vi "ReversedEngineering GetCompleteDependencyInfo.vi"(1 "path":path[](array[path]), 2 "SearchElements":T2[](array[typedef]), 4 "IgnoreClasses":path[](array[path]), 5 "error in (no error)":errorcluster, 6 "Only Create this class and its dependencis":bool, 7 "SyncOption":T1, 8 "Only analyse this class methods and attributes(False)":bool, 10 "CreateApplicationNode":bool) -> (15 "classInfos":T7[](array[typedef]), 16 "TypeDefs":T3[](array[typedef]), 17 "Cancelled":bool, 19 "error out":errorcluster)   [LabVIEW 2014]
doc: "Gets current diagram values"
uses:
  <resource>/Framework/Providers/Open_GDS/UML/ReversedEngineering/ReversedEngineering ClassInfoType.ctl
  <resource>/Framework/Providers/Open_GDS/UML/UMLEditor/UMLEditor_VisibilityType.ctl
  <resource>/Framework/Providers/Open_GDS/UML/ReversedEngineering/ReversedEngineering AttributeInfoType.ctl
  <resource>/Framework/Providers/Open_GDS/ClassProviders/Common/CommonVIs/CommonVIs_AttributeDataType.ctl
  <resource>/Framework/Providers/Open_GDS/UML/ReversedEngineering/ReversedEngineering_ClassDependencyDetailsType.ctl
  <resource>/Framework/Providers/Open_GDS/ClassProviders/Common/ScriptingFunctions/SubVIs/Scripting_ViDependencyType.ctl
  <resource>/Framework/Providers/Open_GDS/UML/ReversedEngineering/ReversedEngineering TypeDefType.ctl
  <resource>/Framework/Providers/Open_GDS/UML/ReversedEngineering/ReversedEngineering RecursiveSearchElements.ctl
  <resource>/Framework/Providers/Open_GDS/UML/UMLEditor/UMLEditor_SyncOptions.ctl
  <resource>/Framework/Providers/Open_GDS/UML/UMLEditor/UMLEditor BusyDialogAction.ctl
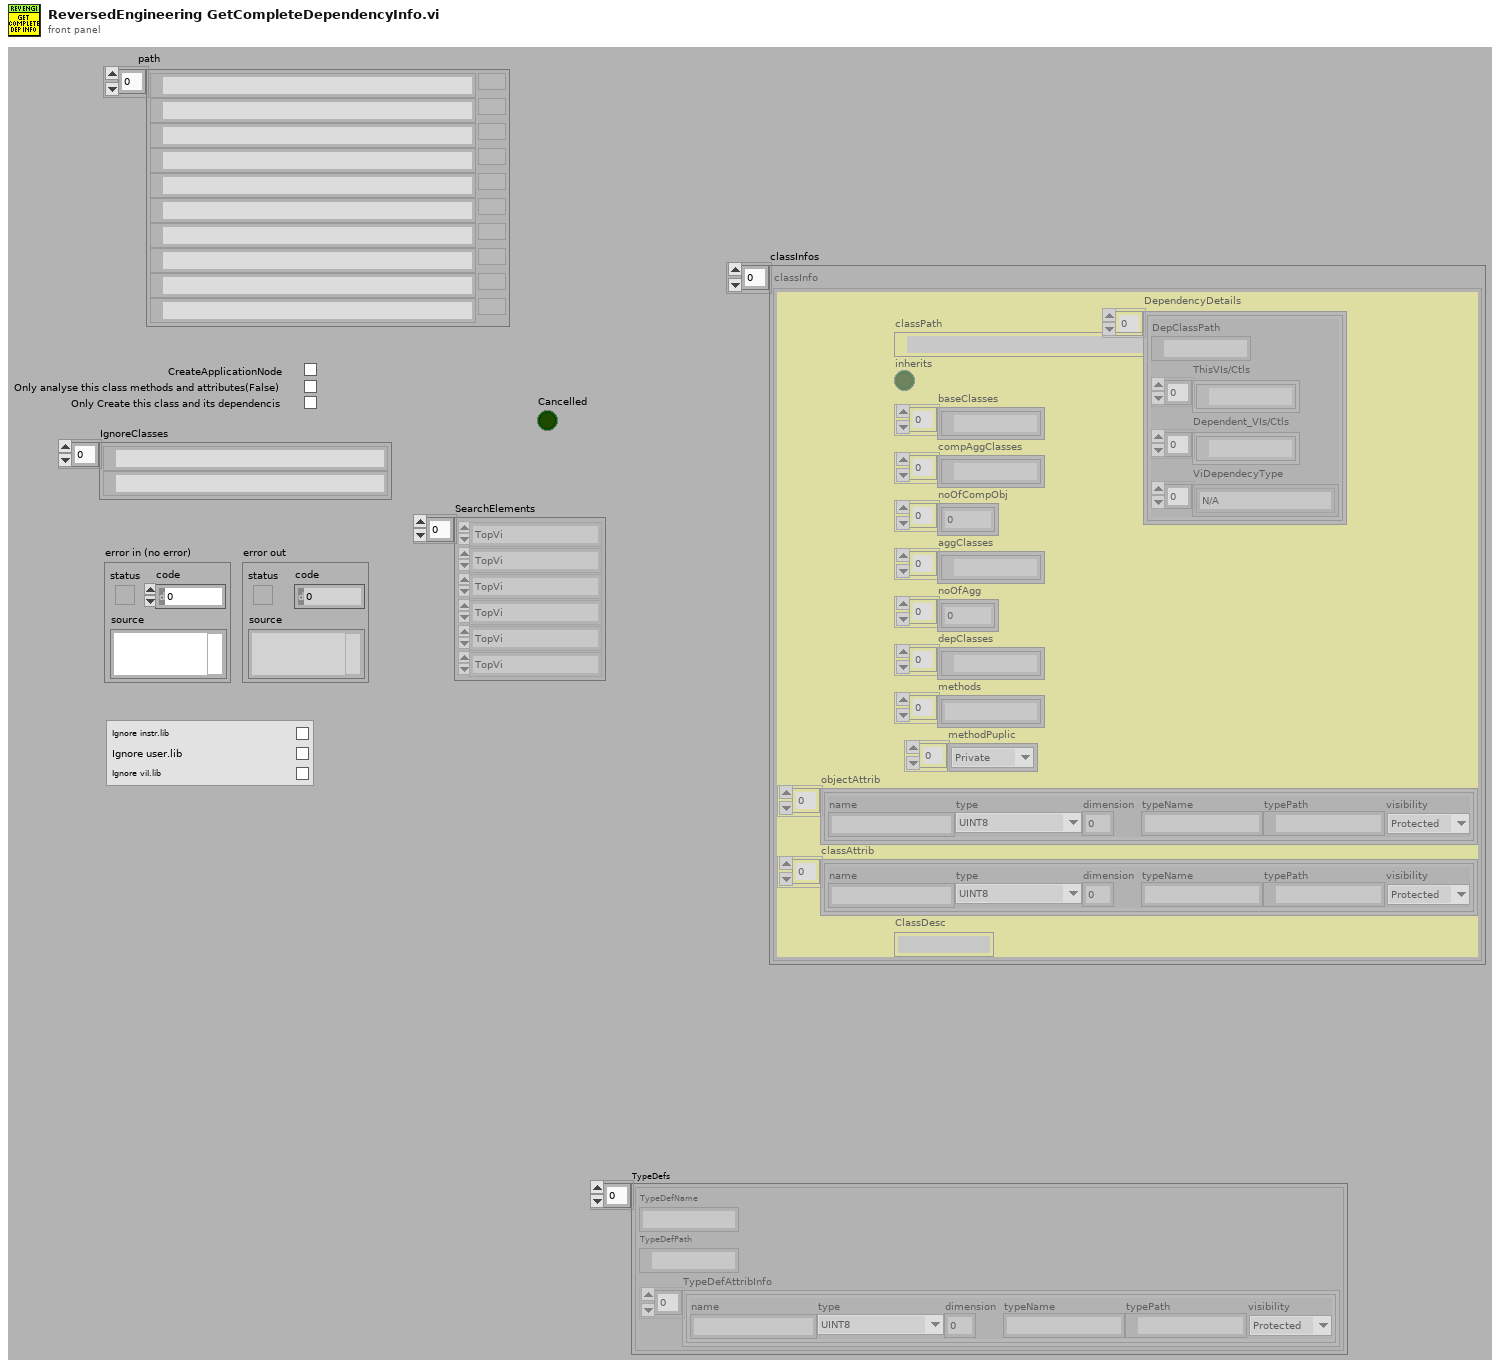
[diagram p1: front panel]
types:
  T1 = typedef "UMLEditor_SyncOptions.ctl" = cluster{"IgnoreInstrLib":bool, "IgnoreUserLib":bool, "IgnoreViLib":bool}
  T2 = typedef "ReversedEngineering RecursiveSearchElements.ctl" = enum16{"TopVi", "Class", "Dir", "Dir(rec.)"}
  T3 = typedef "ReversedEngineering TypeDefType.ctl" = cluster{"TypeDefName":string, "TypeDefPath":path, "TypeDefAttribInfo":T4[]}
  T4 = typedef "ReversedEngineering AttributeInfoType.ctl" = cluster{"name":string, "type":T5, "dimension":i32, "typeName":string, "typePath":path, "visibility":T6}
  T5 = typedef "CommonVIs_AttributeDataType.ctl" = enum16{"UINT8", "INT8", "UINT16", "INT16", "UINT32", "INT32", "UINT64", "INT64", "SGL", "DBL", "EXT", "CSG", "CDB", "CXT", "TimeStamp", "STRING", "PATH", "BOOL", "ENUM", "RefNum", "VIRefNum", "LabVIEW Class", "Cluster", "Variant", "TypeDef", "Waveform", "LabVIEW Object", "Other", "void"}
  T6 = typedef "UMLEditor_VisibilityType.ctl" = enum16{"Public", "Private", "Protected"}
  T7 = typedef "ReversedEngineering ClassInfoType.ctl" = cluster{"classPath":path, "inherits":bool, "baseClasses":path[], "compAggClasses":path[], "noOfCompObj":i32[], "aggClasses":path[], "noOfAgg":i32[], "depClasses":path[], "methods":string[], "methodPuplic":T6[], "objectAttrib":T4[], "classAttrib":T4[], "ClassDesc":string, "DependencyDetails":T8[]}
  T8 = typedef "ReversedEngineering_ClassDependencyDetailsType.ctl" = cluster{"DepClassPath":path, "ThisVIs/Ctls":path[], "Dependent_VIs/Ctls":path[], "ViDependecyType":T9[]}
  T9 = typedef "Scripting_ViDependencyType.ctl" = enum16{"N/A", "Launches"}
  T10 = cluster{"dependencyClassPath":path[], "topVIPath":path, "classInfos":T7[], "calleesVIs":path[], "VIRef":refnum<vi>[], "TypeDefs":T3[], "TopVIPath":path, "SearchOnlyClasses":bool, "SearchDirs":path[], "SearchOnlyTopVIs":bool, "lvclasses":path[]}
  T11 = enum16{"Get Library Info", "Create Library Info", "Clear Library Info"}
  T12 = typedef "UMLEditor BusyDialogAction.ctl" = enum16{"Initialize", "Open(VIs)", "Open(i)", "Send_I-Value", "SendStatusMessage", "GetBusyDialogStatus", "Close", "Quit"}
  T13 = typedef "Librarian File Info Out.ctl" = cluster{"creation date":u32, "last mod date":u32, "type":string, "creator":string, "LV version":i32, "size":i32, "top level":bool}
  T14 = typedef "Scripting_VIClassDependency.ctl" = cluster{"VIPath":path, "Class":string, "ClassPath":path, "ViDependencyType":T9}
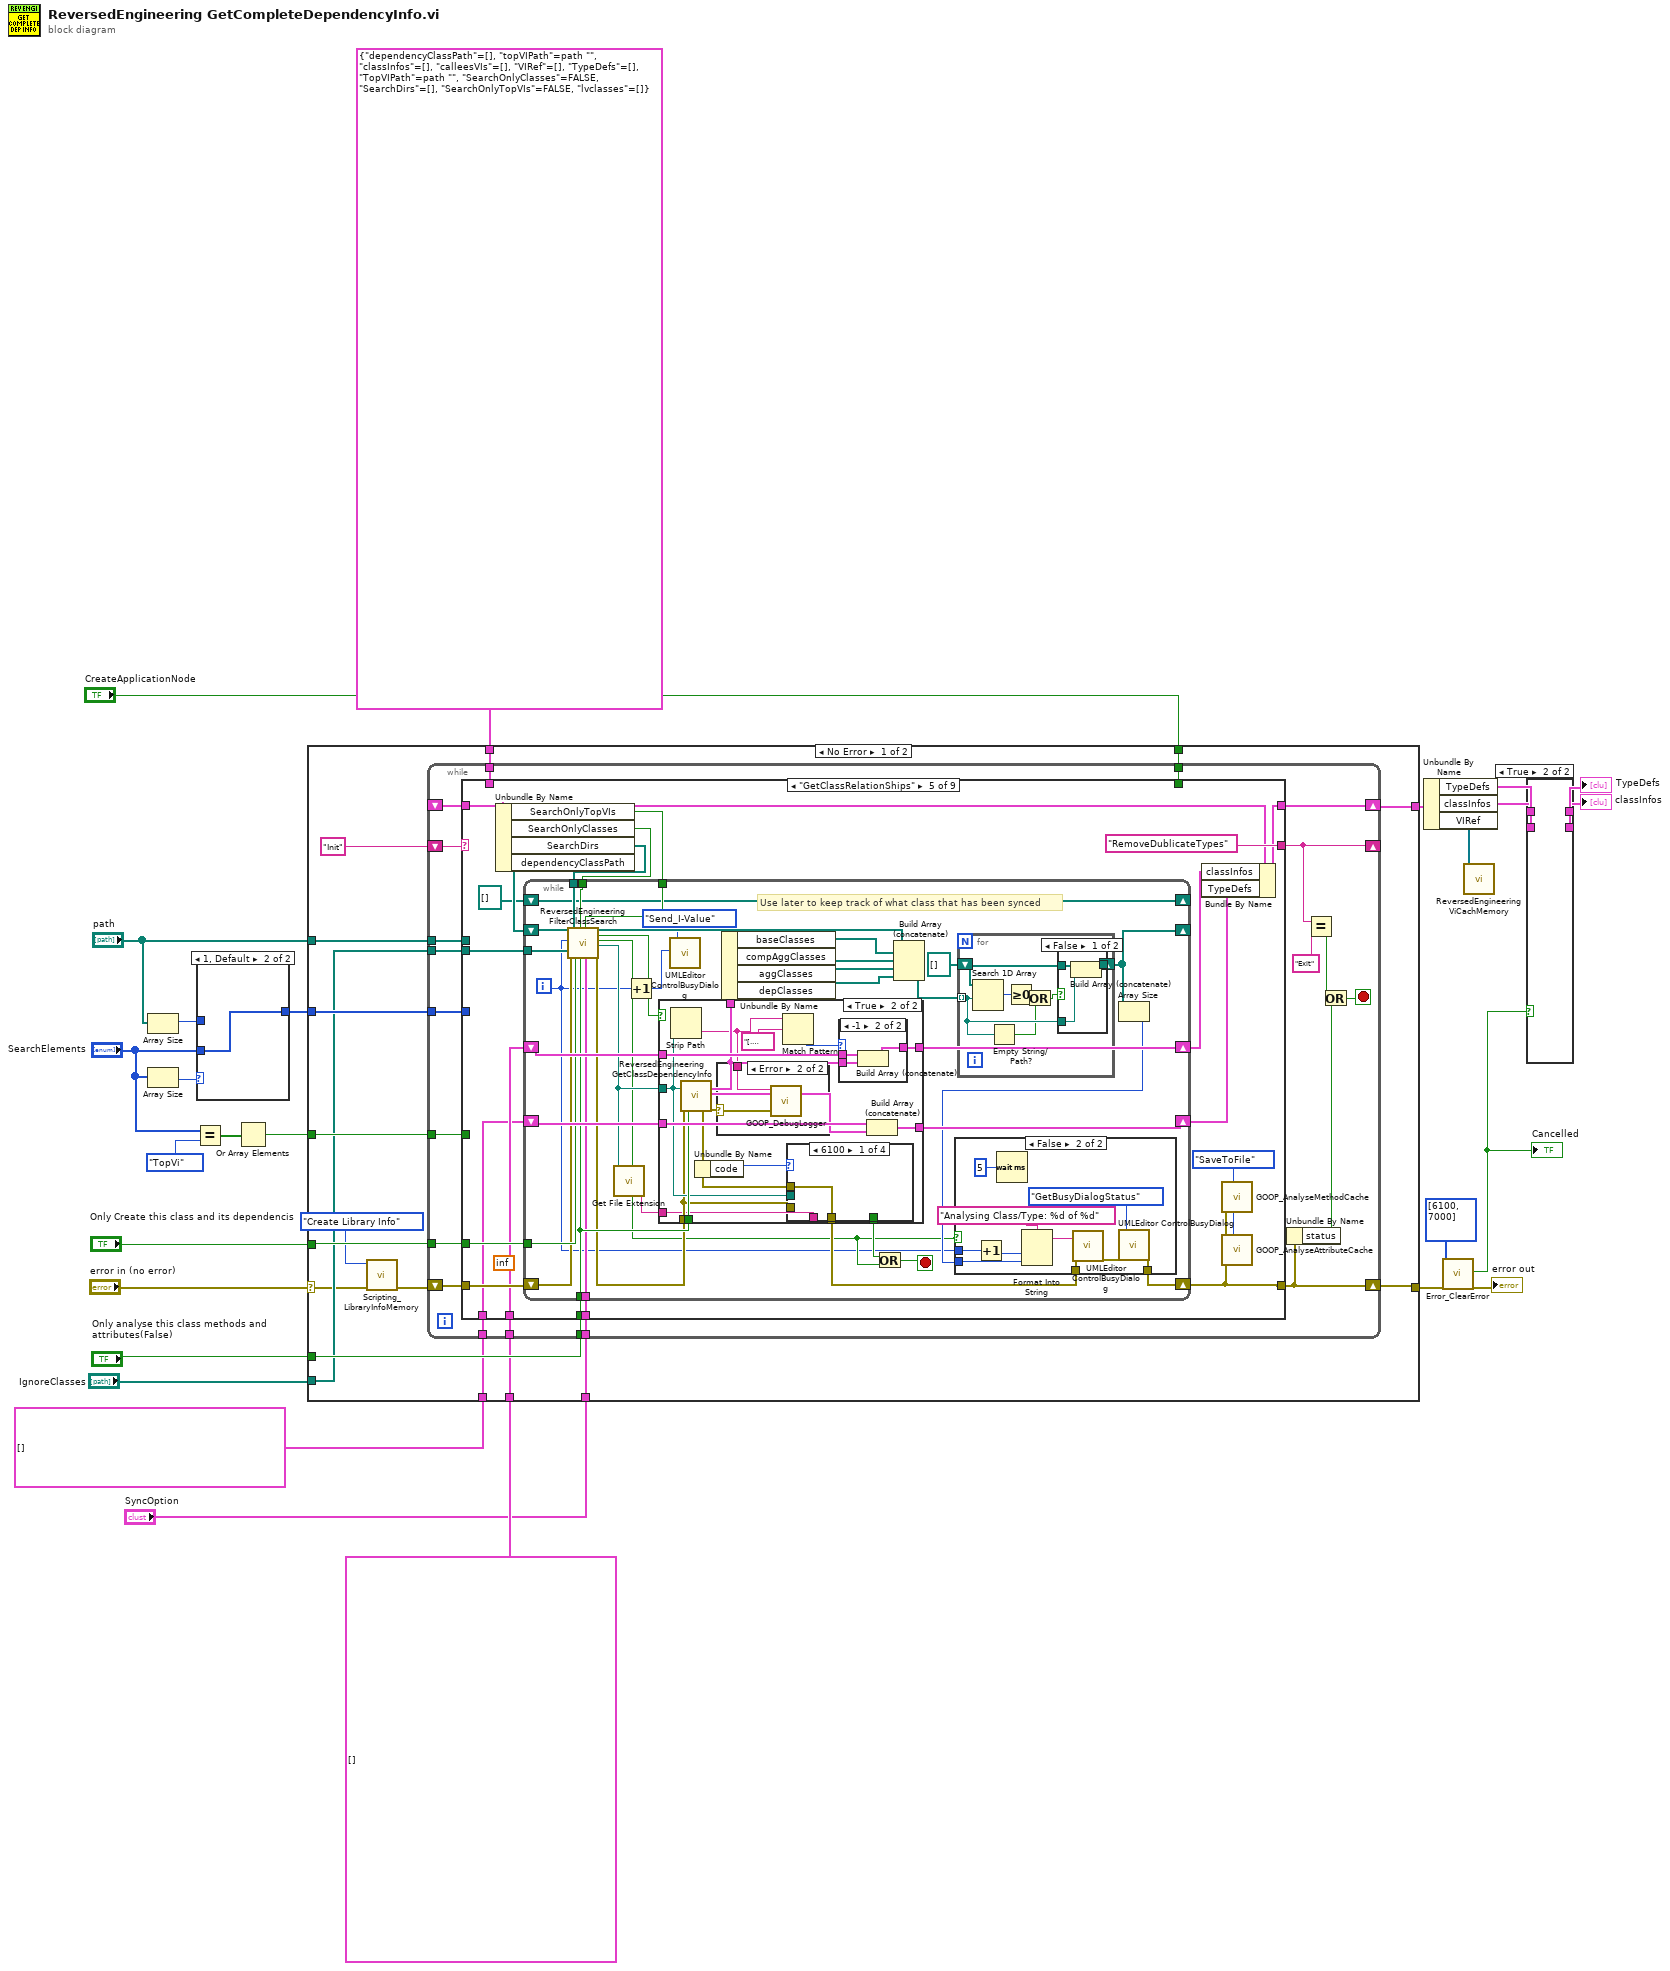
[diagram p0: block diagram]
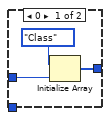
[diagram p3: hidden frame]
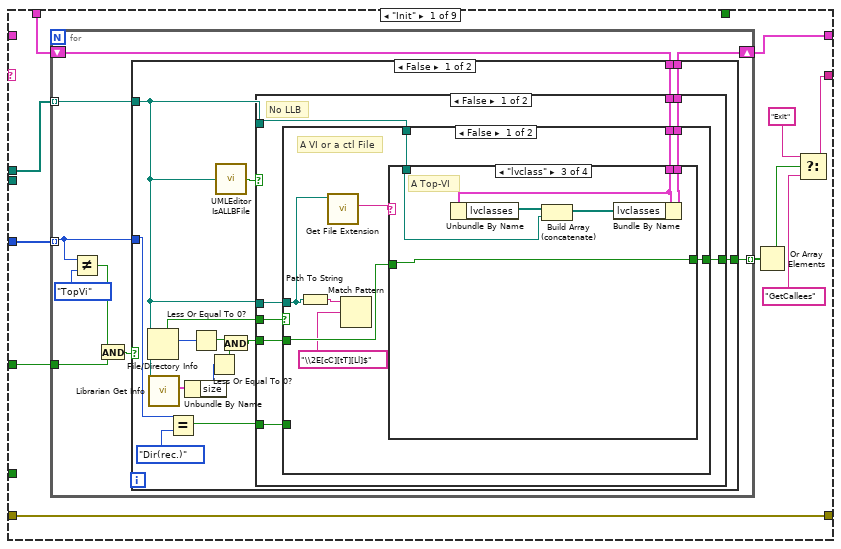
[diagram p4: hidden frame]
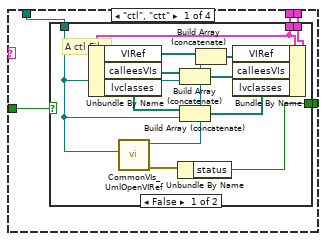
[diagram p5: hidden frame]
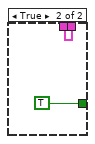
[diagram p6: hidden frame]
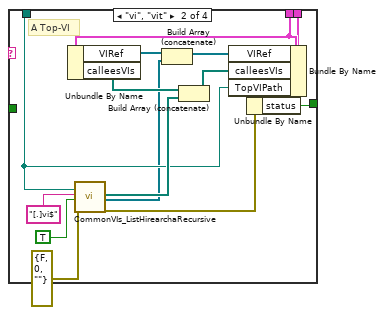
[diagram p7: hidden frame]
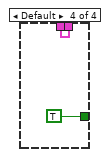
[diagram p8: hidden frame]
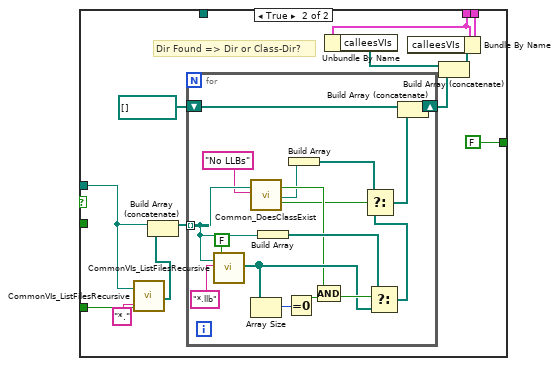
[diagram p9: hidden frame]
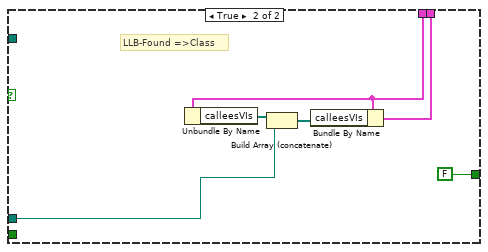
[diagram p10: hidden frame]
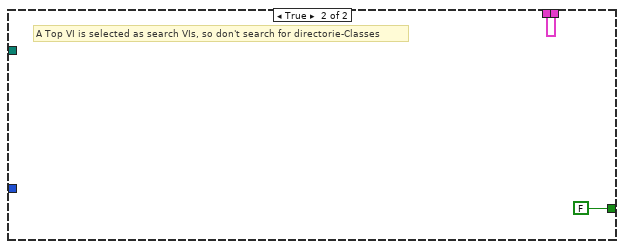
[diagram p11: hidden frame]
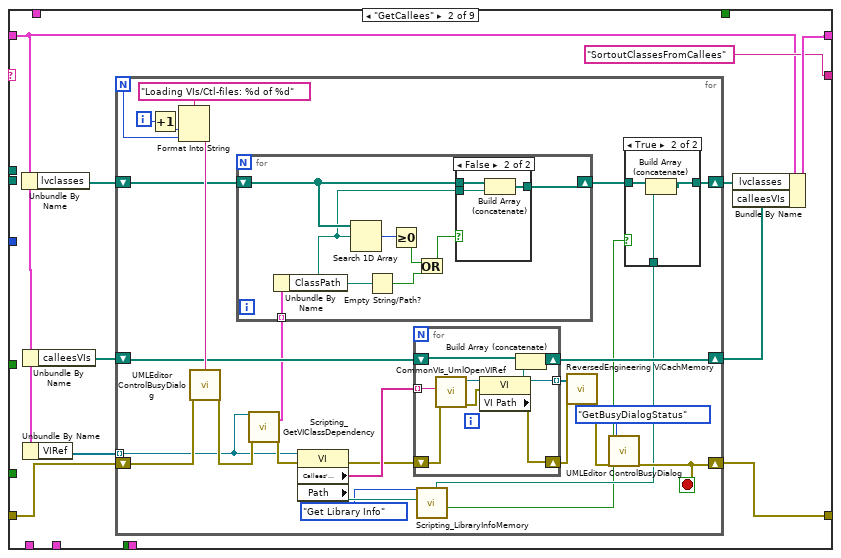
[diagram p12: hidden frame]
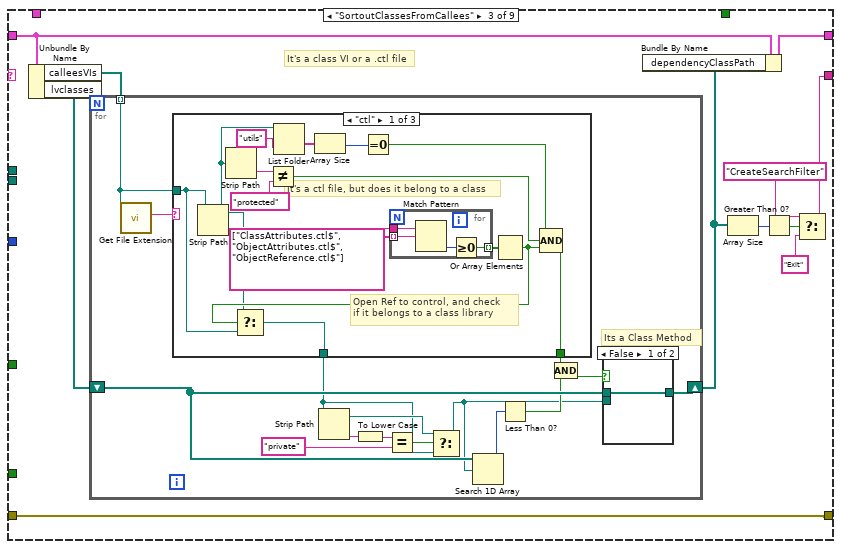
[diagram p15: hidden frame]
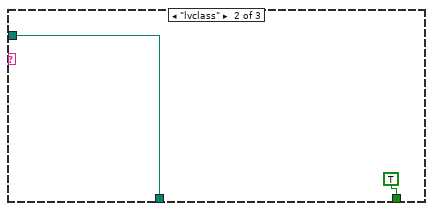
[diagram p16: hidden frame]
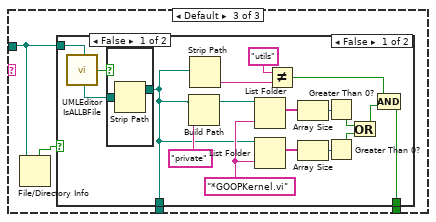
[diagram p17: hidden frame]
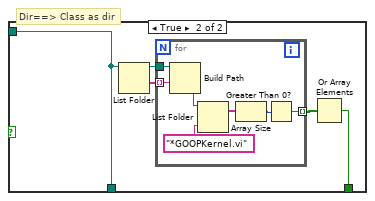
[diagram p19: hidden frame]
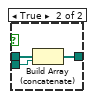
[diagram p20: hidden frame]
diagram:
  n1 = Array Size(array="path") -> (size(s)=w19:i32)
  n2 = Array Size(array="SearchElements") -> (size(s)=w21:i32)
  n3 = Equal?(x="SearchElements", y=ReversedEngineering_RecursiveSearchElements."TopVi" ("Enum")) -> (x = y?=w9:bool[])
  n4 = case shown="1, Default" w21 {
    tunnel: w19 -> [w29 _]
    tunnel: [w28 w31] -> w18
    tunnel: "SearchElements" -> [_ w31]
    frame 0 {
      n5 = Initialize Array(ReversedEngineering_RecursiveSearchElements."Class" ("Enum"), w29) -> (w28:T2[])
    }
    frame 1, Default {
    }
  }
  n6 = Or Array Elements(Boolean array=w9) -> (logical OR=w7:bool)
  n7 = case shown="No Error" "error in (no error)" {
    selector: "error in (no error)" -> [w34 w634]
    tunnel: [w47 w634] -> w17
    tunnel: "path" -> [w46 _]
    tunnel: [w45 _] -> w26
    tunnel: "Only Create this class and its dependencis" -> [w44 _]
    tunnel: "Only analyse this class methods and attributes(False)" -> [w41 _]
    tunnel: "CreateApplicationNode" -> [w43 _]
    tunnel: w18 -> [w42 _]
    tunnel: w7 -> [w40 _]
    tunnel: T10 {"dependencyClassPath"=[], "topVIPath"=path "", "classInfos"=[], "calleesVIs"=[], "VIRef"=[], "TypeDefs"=[], "TopVIPath"=path "", "SearchOnlyClasses"=FALSE, "SearchDirs"=[], "SearchOnlyTopVIs"=FALSE, "lvclasses"=[]} ("Cluster") -> [w39 _]
    tunnel: T7[] [] -> [w38 _]
    tunnel: T3[] [] -> [w37 _]
    tunnel: "IgnoreClasses" -> [w36 _]
    tunnel: "SyncOption" -> [w35 _]
    frame No Error {
      n8 = call <resource>:"Scripting_LibraryInfoMemory.vi"("error in (no error)"=w34, "Action"=T11."Create Library Info") -> ("error out"=w33:errorcluster)  [unwired: 5 in, 4 out]
      n9 = while {
        shift-right: [w66] -> _
        shift-left: "Init" -> [w69]
        shift-right: [w67] -> w47
        shift-left: w33 -> [w68]
        shift-right: [w60] -> w45
        shift-left: _ -> [w61]
        tunnel: w46 -> [w59]
        tunnel: w44 -> [w58]
        tunnel: w43 -> [w57]
        tunnel: w42 -> [w56]
        tunnel: w41 -> [w55]
        tunnel: w40 -> [w54]
        tunnel: w39 -> [w53]
        tunnel: w38 -> [w52]
        tunnel: w37 -> [w51]
        tunnel: w36 -> [w50]
        tunnel: w35 -> [w49]
        stop <- w62 stop-if-true
        n10 = case shown="\"GetClassRelationShips\"" w69 {
          tunnel: w68 -> [w80 w205 w269 w351 w416 w522 w553 w623 w631]
          tunnel: [w80 w206 w269 w348 w402 w522 w553 w623 w631] -> w67
          tunnel: [w79 "SortoutClassesFromCallees" ("y") w264 "GetClassRelationShips" ("y") "RemoveDublicateTypes" ("y") "RemoveClassDependenciesDueToInheritance" ("y") w549 "Exit" ("y") "Exit" ("y")] -> w66
          tunnel: w61 -> [_ w202 w268 w363 w417 w525 w555 w622 w633]
          tunnel: [w73 w208 w270 w362 w418 w523 w554 w621 w633] -> w60
          tunnel: w59 -> [w78 _ _ w358 _ _ _ _ _]
          tunnel: w58 -> [_ _ _ _ w413 _ _ _ _]
          tunnel: w57 -> [_ _ _ _ _ _ w547 _ _]
          tunnel: w56 -> [w72 _ _ w353 _ _ _ _ _]
          tunnel: w55 -> [_ _ _ _ w411 _ _ _ _]
          tunnel: w54 -> [w71 _ _ _ _ _ _ _ _]
          tunnel: w53 -> [w70 _ _ _ _ _ _ _ _]
          tunnel: w52 -> [_ _ _ _ w407 _ _ _ _]
          tunnel: w51 -> [_ _ _ _ w406 _ _ _ _]
          tunnel: w50 -> [_ _ _ _ w404 _ _ _ _]
          tunnel: w49 -> [_ _ _ _ w403 _ _ _ _]
          frame "Init" {
            n11 = for {
              tunnel: w78 -> [w86] mode=indexing
              shift-right: [w88] -> w73
              shift-left: w70 -> [w89]
              tunnel: [w87] -> w77 mode=indexing
              tunnel: w72 -> [w85] mode=indexing
              tunnel: w71 -> [w81]
              n12 = Not Equal?(x=w85, y=ReversedEngineering_RecursiveSearchElements."TopVi") -> (x != y?=w83:bool)
              n13 = And(x=w83, y=w81) -> (x .and. y?=w82:bool)
              n14 = case shown="False" w82 {
                tunnel: w89 -> [w104 w198]
                tunnel: [w103 w198] -> w88
                tunnel: [w102 FALSE ("status")] -> w87
                tunnel: w86 -> [w94 _]
                tunnel: w85 -> [w97 _]
                frame False {
                  n15 = File/Directory Info(path=w94) -> (directory=w100:bool, size=w96:i64)  [unwired: 1 in, 5 out]
                  n16 = call <vilib>:"Librarian Get Info.vi"("path"=w94) -> ("file information"=w93:T13)  [unwired: 1 in, 9 out]
                  n17 = Equal?(x=w97, y=ReversedEngineering_RecursiveSearchElements."Dir(rec.)") -> (x = y?=w98:bool)
                  n18 = Unbundle By Name(w93) -> ("size"=w92:i32)
                  n19 = Less Or Equal To 0?(x=w96) -> (x <= 0?=w95:bool)
                  n20 = Less Or Equal To 0?(x=w92) -> (x <= 0?=w91:bool)
                  n21 = call <resource>:"UMLEditor IsALLBFile.vi"("path"=w94) -> ("path to VI library?"=w101:bool)
                  n22 = And(x=w95, y=w91) -> (x .and. y?=w90:bool)
                  n23 = case shown="False" w101 {
                    tunnel: w90 -> [w112 _]
                    tunnel: w94 -> [w111 _]
                    tunnel: w104 -> [w110 w194]
                    tunnel: [w109 w195] -> w103
                    tunnel: [w108 FALSE ("status")] -> w102
                    tunnel: w94 -> [w106 w193]
                    tunnel: w100 -> [w107 _]
                    tunnel: w98 -> [w105 _]
                    frame False {
                      # "No LLB"
                      n24 = case shown="False" w107 {
                        tunnel: w112 -> [w121 _]
                        tunnel: w111 -> [w120 _]
                        tunnel: w110 -> [w119 w172]
                        tunnel: [w118 w171] -> w109
                        tunnel: [w117 FALSE] -> w108
                        tunnel: w106 -> [w114 w167]
                        tunnel: w105 -> [_ w168]
                        frame False {
                          # "A VI or a ctl File"
                          n25 = Path To String(path=w114) -> (string=w116:string)
                          n26 = call <vilib>:"Get File Extension.vi"("file"=w114) -> ("lowercase file extension"=w113:string)  [unwired: 1 in, 9 out]
                          n27 = Match Pattern(string=w116, regular expression="\\2E[cC][tT][Ll]$") -> ()  [unwired: 5 out]
                          n28 = case shown="\"lvclass\"" w113 {
                            tunnel: w121 -> [w126 _ w155 _]
                            tunnel: w120 -> [w125 w143 w156 _]
                            tunnel: w119 -> [w124 w152 w158 w162]
                            tunnel: [w123 w151 w157 w162] -> w118
                            tunnel: [w122 w148 w155 TRUE ("status")] -> w117
                            frame "ctl", "ctt" {
                              n29 = case shown="False" w126 {
                                tunnel: w125 -> [w127 _]
                                tunnel: w124 -> [w134 w140]
                                tunnel: [w136 w140] -> w123
                                tunnel: [w132 TRUE] -> w122
                                frame False {
                                # "A ctl File"
                                n30 = Unbundle By Name(w134) -> ("VIRef"=w137:refnum<vi>[], "calleesVIs"=w131:path[], "lvclasses"=w129:path[])
                                n31 = call <resource>:"CommonVIs_UmlOpenVIRef.vi"("ViPath/ViName"=w127) -> ("error out"=w133:errorcluster, "vi reference"=w135:refnum<vi>)  [unwired: 3 in, 6 out]
                                n32 = Unbundle By Name(w133) -> ("status"=w132:bool)
                                n33 = Build Array (concatenate)(w131, w127) -> (w130:path[])
                                n34 = Build Array (concatenate)(w129, w127) -> (w128:path[])
                                n35 = Build Array (concatenate)(w137, w135) -> (w138:refnum<vi>[])
                                n36 = Bundle By Name(cluster=w134, "VIRef"=w138, "calleesVIs"=w130, "lvclasses"=w128) -> (w136:T10)
                                }
                                frame True {
                                }
                              }
                            }
                            frame "vi", "vit" {
                              # "A Top-VI"
                              n37 = Unbundle By Name(w152) -> ("VIRef"=w153:refnum<vi>[], "calleesVIs"=w150:path[])
                              n38 = call <resource>:"CommonVIs_ListHirearchaRecursive.vi"("FilePath"=w143, "FileSearchPattern"="[.]vi$", "IgnoreClassMemberVIs(False)"=TRUE ("IgnoreClassMemberVIs(Flase)"), "error in (no error)"=errorcluster {"status"=FALSE, "code"=0, "source"=""}) -> ("Files"=w145:path[], "VIRefs"=w142:refnum<vi>[], "error out"=w144:errorcluster)  [unwired: 13 out]
                              n39 = Build Array (concatenate)(w153, w142) -> (w154:refnum<vi>[])
                              n40 = Build Array (concatenate)(w150, w145) -> (w149:path[])
                              n41 = Bundle By Name(cluster=w152, "VIRef"=w154, "calleesVIs"=w149, "TopVIPath"=w143) -> (w151:T10)
                              n42 = Unbundle By Name(w144) -> ("status"=w148:bool)
                            }
                            frame "lvclass" {
                              # "A Top-VI"
                              n43 = Unbundle By Name(w158) -> ("lvclasses"=w159:path[])
                              n44 = Build Array (concatenate)(w159, w156) -> (w160:path[])
                              n45 = Bundle By Name(cluster=w158, "lvclasses"=w160) -> (w157:T10)
                            }
                            frame Default {
                            }
                          }
                        }
                        frame True {
                          # "Dir Found => Dir or Class-Dir?"
                          n46 = call <resource>:"CommonVIs_ListFilesRecursive.vi"("directory path"=w167, "FileSearchPattern"="*." ("pattern"), "RecusiveSearch(True)"=w168) -> ("Directories"=w166:path[])  [unwired: 3 in, 13 out]
                          n47 = Build Array (concatenate)(w167, w166) -> (w165:path[])
                          n48 = for {
                            tunnel: w165 -> [w182] mode=indexing
                            shift-right: [w187] -> w163
                            shift-left: path[] [] ("calleesVIs") -> [w186]
                            n49 = call <resource>:"CommonVIs_ListFilesRecursive.vi"("directory path"=w182, "FileSearchPattern"="*.llb" ("pattern"), "RecusiveSearch(True)"=FALSE ("RecusiveSerach(True)")) -> ("Files"=w184:path[])  [unwired: 3 in, 13 out]
                            n50 = call <resource>:"Common_DoesClassExist.vi"("ClassPath"=w182, "ClassName"="No LLBs") -> ("ClassExists"=w181:bool, "llb/LvCLass-Path"=w179:path, "LvClassExists"=w178:bool)  [unwired: 15 out]
                            n51 = Array Size(array=w184) -> (size(s)=w191:i32)
                            n52 = Build Array(w182) -> (w183:path[])
                            n53 = Equal To 0?(x=w191) -> (x = 0?=w190:bool)
                            n54 = Build Array(w179) -> (w177:path[])
                            n55 = Compound Arithmetic op=AND(w181, w190) -> (w185:bool)
                            n56 = Select(t=w183, s=w185, f=w184) -> (s? t:f=w175:path[])
                            n57 = Select(t=w177, s=w178, f=w175) -> (s? t:f=w176:path[])
                            n58 = Build Array (concatenate)(w186, w176) -> (w187:path[])
                          }
                          n59 = Unbundle By Name(w172) -> ("calleesVIs"=w174:path[])
                          n60 = Build Array (concatenate)(w174, w163) -> (w173:path[])
                          n61 = Bundle By Name(cluster=w172, "calleesVIs"=w173) -> (w171:T10)
                        }
                      }
                    }
                    frame True {
                      # "LLB-Found =>Class"
                      n62 = Unbundle By Name(w194) -> ("calleesVIs"=w197:path[])
                      n63 = Build Array (concatenate)(w197, w193) -> (w196:path[])
                      n64 = Bundle By Name(cluster=w194, "calleesVIs"=w196) -> (w195:T10)
                    }
                  }
                }
                frame True {
                  # "A Top VI is selected as search VIs, so don't search for directorie-Classes"
                }
              }
            }
            n65 = Or Array Elements(Boolean array=w77) -> (logical OR=w76:bool)
            n66 = Select(t="Exit", s=w76, f="GetCallees") -> (s? t:f=w79:string)
          }
          frame "GetCallees" {
            n67 = Unbundle By Name(w202) -> ("lvclasses"=w201:path[])
            n68 = Unbundle By Name(w202) -> ("calleesVIs"=w203:path[])
            n69 = Unbundle By Name(w202) -> ("VIRef"=w209:refnum<vi>[])
            n70 = for {
              N -> [w230]
              tunnel: w209 -> [w214] mode=indexing
              shift-right: [w234] -> w204
              shift-left: w203 -> [w224]
              shift-right: [w217] -> w206
              shift-left: w205 -> [w216]
              shift-right: [w218] -> w200
              shift-left: w201 -> [w221]
              i -> [w232]
              stop <- w217 stop-if-true
              n71 = Increment(x=w232) -> (x+1=w231:i32)
              n72 = Format Into String(format string="Loading VIs/Ctl-files: %d of %d", w231, w230) -> (resulting string=w229:string)  [unwired: 2 in, 1 out]
              n73 = call <resource>:"UMLEditor ControlBusyDialog.vi"("Title/StatusText"=w229, "error in (no error)"=w216) -> ("error out"=w215:errorcluster)  [unwired: 2 in, 15 out]
              n74 = call <resource>:"Scripting_GetVIClassDependency.vi"("ViRef"=w214, "error in (no error)"=w215) -> ("DepVIs"=w222:T14[], "error out"=w223:errorcluster)  [unwired: 16 out]
              n75 = for {
                tunnel: w222 -> [w246] mode=indexing
                shift-right: [w247] -> w219
                shift-left: w221 -> [w245]
                n76 = Unbundle By Name(w246) -> ("ClassPath"=w243:path)
                n77 = Search 1D Array(1D array=w245, element=w243) -> (index of element=w244:i32)  [unwired: 1 out]
                n78 = Empty String/Path?(string/path=w243) -> (empty?=w241:bool)
                n79 = Greater Or Equal To 0?(x=w244) -> (x >= 0?=w242:bool)
                n80 = Or(x=w242, y=w241) -> (x .or. y?=w240:bool)
                n81 = case shown="False" w240 {
                  tunnel: w245 -> [w248 w251]
                  tunnel: [w248 w250] -> w247
                  tunnel: w243 -> [_ w249]
                  frame True {
                  }
                  frame False {
                    n82 = Build Array (concatenate)(w251, w249) -> (w250:path[])
                  }
                }
              }
              n83 = property class="VI"(reference=w214, error in=w223) -> (error out=w220:errorcluster, "Callees' Names"=w235:string[], "Path"=w213:path)  [unwired: 1 out]
              n84 = for {
                tunnel: w235 -> [w254] mode=indexing
                shift-right: [w258] -> w234
                shift-left: w224 -> [w260]
                shift-right: [w253] -> w226
                shift-left: w220 -> [w259]
                tunnel: [w252] -> w227 mode=indexing
                n85 = call <resource>:"CommonVIs_UmlOpenVIRef.vi"("error in"=w259, "ViPath/ViName"=w254) -> ("error out"=w256:errorcluster, "vi reference"=w257:refnum<vi>)  [unwired: 2 in, 6 out]
                n86 = property class="VI"(reference=w257, error in=w256) -> (reference out=w252:refnum<vi>, error out=w253:errorcluster, "VI Path"=w255:path)
                n87 = Build Array (concatenate)(w260, w255) -> (w258:path[])
              }
              n88 = call <resource>:"Scripting_LibraryInfoMemory.vi"("ViPath"=w213, "Action"=T11."Get Library Info") -> ("Found"=w211:bool, "LibaryPath"=w212:path)  [unwired: 5 in, 3 out]
              n89 = call <resource>:"ReversedEngineering ViCachMemory.vi"("ViRef-Array"=w227, "error in (no error)"=w226) -> ("error out"=w225:errorcluster)  [unwired: 2 in, 15 out]
              n90 = call <resource>:"UMLEditor ControlBusyDialog.vi"("error in (no error)"=w225, "Action(SendStatusMessage)"=UMLEditor_BusyDialogAction."GetBusyDialogStatus") -> ("error out"=w217:errorcluster)  [unwired: 2 in, 15 out]
              n91 = case shown="True" w211 {
                tunnel: w219 -> [w236 w239]
                tunnel: w212 -> [_ w238]
                tunnel: [w236 w237] -> w218
                frame False {
                }
                frame True {
                  n92 = Build Array (concatenate)(w239, w238) -> (w237:path[])
                }
              }
            }
            n93 = Bundle By Name(cluster=w202, "lvclasses"=w200, "calleesVIs"=w204) -> (w208:T10)
          }
          frame "SortoutClassesFromCallees" {
            # "It's a class VI or a .ctl file"
            n94 = Unbundle By Name(w268) -> ("calleesVIs"=w271:path[], "lvclasses"=w261:path[])
            n95 = for {
              tunnel: w271 -> [w273] mode=indexing
              shift-right: [w284] -> w267
              shift-left: w261 -> [w285]
              # "Its a Class Method"
              n96 = call <vilib>:"Get File Extension.vi"("file"=w273) -> ("lowercase file extension"=w272:string)  [unwired: 1 in, 9 out]
              n97 = case shown="\"ctl\"" w272 {
                tunnel: [w293 TRUE w311] -> w281
                tunnel: [w301 w307 w310] -> w274
                tunnel: w273 -> [w297 w307 w308]
                frame "ctl" {
                  # "Open Ref to control, and check\nif it belongs to a class library"
                  # "It's a ctl file, but does it belong to a class"
                  n98 = Strip Path(path=w297) -> (stripped path=w291:path, name=w300:string)
                  n99 = Strip Path(path=w291) -> (name=w296:string)  [unwired: 1 out]
                  n100 = Not Equal?(x=w296, y="protected") -> (x != y?=w292:bool)
                  n101 = List Folder(path=w291, pattern="utils" ("y")) -> (folder names=w290:string[])  [unwired: 1 in, 4 out]
                  n102 = Array Size(array=w290) -> (size(s)=w288:i32)
                  n103 = Equal To 0?(x=w288) -> (x = 0?=w287:bool)
                  n104 = for {
                    tunnel: w300 -> [w305]
                    tunnel: string[] ["ClassAttributes.ctl$", "ObjectAttributes.ctl$", "ObjectReference.ctl$"] -> [w304] mode=indexing
                    tunnel: [w302] -> w298 mode=indexing
                    n105 = Match Pattern(string=w305, regular expression=w304) -> (offset past match=w303:i32)  [unwired: 4 out]
                    n106 = Greater Or Equal To 0?(x=w303) -> (x >= 0?=w302:bool)
                  }
                  n107 = Or Array Elements(Boolean array=w298) -> (logical OR=w294:bool)
                  n108 = Select(t=w291, s=w294, f=w297) -> (s? t:f=w301:path)
                  n109 = Compound Arithmetic op=AND(w287, w292, w294) -> (w293:bool)
                }
                frame "lvclass" {
                }
                frame Default {
                  n110 = File/Directory Info(path=w308) -> (directory=w309:bool)  [unwired: 1 in, 6 out]
                  n111 = case shown="False" w309 {
                    tunnel: [w312 w332] -> w311
                    tunnel: [w317 w336] -> w310
                    tunnel: w308 -> [w324 w336]
                    frame False {
                      w319 = "*GOOPKernel.vi" ("pattern")
                      n112 = call <resource>:"UMLEditor IsALLBFile.vi"("path"=w324) -> ("path to VI library?"=w328:bool)
                      n113 = case shown="False" w328 {
                        tunnel: [w330 w331] -> w317
                        tunnel: w324 -> [w329 w331]
                        frame False {
                          n114 = Strip Path(path=w329) -> (stripped path=w330:path)  [unwired: 1 out]
                        }
                        frame True {
                        }
                      }
                      n115 = Build Path(base path=w317, name or relative path="private") -> (appended path=w318:path)
                      n116 = Strip Path(path=w317) -> (name=w316:string)  [unwired: 1 out]
                      n117 = List Folder(path=w318, pattern=w319) -> (filenames=w323:string[])  [unwired: 1 in, 4 out]
                      n118 = List Folder(path=w317, pattern=w319) -> (filenames=w326:string[])  [unwired: 1 in, 4 out]
                      n119 = Not Equal?(x="utils" ("name or relative path"), y=w316) -> (x != y?=w314:bool)
                      n120 = Array Size(array=w323) -> (size(s)=w322:i32)
                      n121 = Array Size(array=w326) -> (size(s)=w327:i32)
                      n122 = Greater Than 0?(x=w322) -> (x > 0?=w321:bool)
                      n123 = Greater Than 0?(x=w327) -> (x > 0?=w325:bool)
                      n124 = Or(x=w321, y=w325) -> (x .or. y?=w313:bool)
                      n125 = Compound Arithmetic op=AND(w314, w313) -> (w312:bool)
                    }
                    frame True {
                      # "Dir==> Class as dir"
                      n126 = List Folder(path=w336) -> (path out=w335:path, folder names=w333:string[])  [unwired: 1 in, 4 out]
                      n127 = for {
                        tunnel: w335 -> [w340]
                        tunnel: [w338] -> w334 mode=indexing
                        tunnel: w333 -> [w337] mode=indexing
                        n128 = Build Path(base path=w340, name or relative path=w337) -> (appended path=w339:path)
                        n129 = List Folder(path=w339, pattern="*GOOPKernel.vi") -> (filenames=w342:string[])  [unwired: 1 in, 4 out]
                        n130 = Array Size(array=w342) -> (size(s)=w343:i32)
                        n131 = Greater Than 0?(x=w343) -> (x > 0?=w338:bool)
                      }
                      n132 = Or Array Elements(Boolean array=w334) -> (logical OR=w332:bool)
                    }
                  }
                }
              }
              n133 = Strip Path(path=w274) -> (stripped path=w276:path, name=w280:string)
              n134 = To Lower Case(string=w280) -> (all lower case string=w279:string)
              n135 = Equal?(x=w279, y="private" ("name or relative path")) -> (x = y?=w277:bool)
              n136 = Select(t=w276, s=w277, f=w274) -> (s? t:f=w275:path)
              n137 = Search 1D Array(1D array=w285, element=w275) -> (index of element=w286:i32)  [unwired: 1 out]
              n138 = Less Than 0?(x=w286) -> (x < 0?=w282:bool)
              n139 = Compound Arithmetic op=AND(w281, w282) -> (w283:bool)
              n140 = case shown="False" w283 {
                tunnel: w285 -> [w344 w347]
                tunnel: [w344 w346] -> w284
                tunnel: w275 -> [_ w345]
                frame False {
                }
                frame True {
                  n141 = Build Array (concatenate)(w347, w345) -> (w346:path[])
                }
              }
            }
            n142 = Bundle By Name(cluster=w268, "dependencyClassPath"=w267) -> (w270:T10)
            n143 = Array Size(array=w267) -> (size(s)=w266:i32)
            n144 = Greater Than 0?(x=w266) -> (x > 0?=w265:bool)
            n145 = Select(t="CreateSearchFilter" ("y"), s=w265, f="Exit" ("y")) -> (s? t:f=w264:string)
          }
          frame "CreateSearchFilter" {
            n146 = for {
              tunnel: w353 -> [w368] mode=indexing
              tunnel: w358 -> [w367] mode=indexing
              shift-right: [w369] -> w356
              shift-left: path[] [] -> [w370]
              n147 = case shown="\"Class\"" w368 {
                tunnel: w370 -> [w371 w379 w394 w400]
                tunnel: [w371 w378 w393 w399] -> w369
                tunnel: w367 -> [_ w375 w390 w395]
                frame Default {
                }
                frame "Dir" {
                  n148 = call <resource>:"CommonVIs_ListFilesRecursive.vi"("directory path"=w375, "FileSearchPattern"="*." ("pattern"), "RecusiveSearch(True)"=FALSE ("RecusiveSerach(True)")) -> ("Directories"=w374:path[])  [unwired: 3 in, 13 out]
                  n149 = for {
                    tunnel: w374 -> [w381] mode=indexing
                    shift-right: [w383] -> w372
                    shift-left: path[] [] ("f") -> [w382]
                    n150 = call <resource>:"Common_DoesClassExist.vi"("ClassPath"=w381, "ClassName"="No LLBs") -> ("ClassExists"=w380:bool)  [unwired: 17 out]
                    n151 = case shown="False" w380 {
                      tunnel: [w385 w388] -> w383
                      tunnel: w382 -> [w385 w387]
                      tunnel: w381 -> [_ w386]
                      frame False {
                      }
                      frame True {
                        n152 = Build Array (concatenate)(w387, w386) -> (w388:path[])
                      }
                    }
                  }
                  n153 = Build Array (concatenate)(w379, w375, w372) -> (w378:path[])
                }
                frame "Class" {
                  n154 = File/Directory Info(path=w390) -> (directory=w391:bool)  [unwired: 1 in, 6 out]
                  n155 = Strip Path(path=w390) -> (stripped path=w389:path)  [unwired: 1 out]
                  n156 = Select(t=w390, s=w391, f=w389) -> (s? t:f=w392:path)
                  n157 = Build Array (concatenate)(w394, w392) -> (w393:path[])
                }
                frame "Dir(rec.)" {
                  n158 = call <resource>:"CommonVIs_ListFilesRecursive.vi"("directory path"=w395, "FileSearchPattern"="*.", "SearchInLLBs(True)"=FALSE) -> ("Directories"=w398:path[])  [unwired: 3 in, 13 out]
                  n159 = Build Array (concatenate)(w400, w395, w398) -> (w399:path[])
                }
              }
            }
            n160 = Equal?(x=w353, y=ReversedEngineering_RecursiveSearchElements."TopVi" ("Enum")) -> (x = y?=w355:bool[])
            n161 = Equal?(x=w353, y=ReversedEngineering_RecursiveSearchElements."Class" ("Enum")) -> (x = y?=w360:bool[])
            n162 = And Array Elements(Boolean array=w355) -> (logical AND=w352:bool)
            n163 = And Array Elements(Boolean array=w360) -> (logical AND=w359:bool)
            n164 = Bundle By Name(cluster=w363, "SearchOnlyTopVIs"=w352, "SearchOnlyClasses"=w359, "SearchDirs"=w356) -> (w362:T10)
            n165 = call <resource>:"UMLEditor ControlBusyDialog.vi"("Title/StatusText"="Starts loading VIs", "error in (no error)"=w351) -> ("error out"=w349:errorcluster)  [unwired: 2 in, 15 out]
            n166 = stacked-sequence {
              tunnel: [w366] -> w348
              tunnel: w349 -> [w366]
              frame #0 {
                n167 = Wait (ms)(milliseconds to wait=u32 50) -> ()  [unwired: 1 out]
              }
            }
          }
          frame "GetClassRelationShips" {
            w401 = enum16{"Update", "ReadFromFile", "SaveToFile"}."SaveToFile" ("Actions")
            (unwired) inf
            n168 = Unbundle By Name(w417) -> ("SearchOnlyTopVIs"=w409:bool, "SearchOnlyClasses"=w410:bool, "SearchDirs"=w408:path[], "dependencyClassPath"=w415:path[])
            n169 = while {
              shift-right: [w435] -> w402
              shift-left: w416 -> [w436]
              shift-right: [w434] -> _
              shift-left: w415 -> [w440]
              shift-right: [w448] -> w414
              shift-left: w406 -> [w449]
              tunnel: w413 -> [w441]
              shift-right: [w446] -> w412
              shift-left: w407 -> [w447]
              tunnel: w408 -> [w444]
              tunnel: w410 -> [w443]
              tunnel: w411 -> [w438]
              tunnel: w409 -> [w437]
              shift-right: [w430] -> _
              shift-left: path[] [] -> [w430]
              tunnel: w404 -> [w424]
              tunnel: w403 -> [w423]
              i -> [w421]
              stop <- w426 stop-if-true
              # "Use later to keep track of what class that has been synced"
              n170 = call <resource>:"ReversedEngineering FilterClassSearch.vi"("dependencyClassPath"=w440, "LoopIteration"=w421, "IgnoreClasses"=w424, "error in (no error)"=w436, "SerachDirs"=w444, "Only Create this/these classes and its dependencis"=w441, "SearchOnlyClasses"=w443, "Only analyse this class methods and attributes(False)"=w438, "SearchOnlyTopVIs"=w437, "SyncOption"=w423) -> ("dependencyClassPathOut"=w439:path[], "AnalyseClass"=w442:bool, "AnalyseDone"=w425:bool, "ClassPathToAnalyse"=w429:path, "error out"=w432:errorcluster)  [unwired: 1 in, 4 out]
              n171 = call <vilib>:"Get File Extension.vi"("file"=w429) -> ("filename without extension"=w428:string)  [unwired: 1 in, 9 out]
              n172 = Increment(x=w421) -> (x+1=w420:i32)
              n173 = case shown="True" w442 {
                tunnel: w432 -> [w473 w480]
                tunnel: w449 -> [w474 w492]
                tunnel: [w474 w491] -> w448
                tunnel: w438 -> [_ w489]
                tunnel: w447 -> [w475 w488]
                tunnel: [w475 w487] -> w446
                tunnel: [_ w484] -> w445
                tunnel: w429 -> [_ w483]
                tunnel: [w473 w481] -> w431
                tunnel: w428 -> [_ w479]
                tunnel: [_ w478] -> w427
                frame False {
                }
                frame True {
                  n174 = Strip Path(path=w483) -> (name=w476:string)  [unwired: 1 out]
                  n175 = call <resource>:"ReversedEngineering GetClassDependencyInfo.vi"("Class/Create Path"=w483, "error in (no error)"=w480, "Only analyse this class methods and attributes(False)"=w489) -> ("classInfo"=w484:T7, "TypeDefs"=w490:T3[], "error out"=w477:errorcluster)  [unwired: 14 out]
                  n176 = Unbundle By Name(w477) -> ("code"=w482:i32)
                  n177 = case shown="Error" w477 {
                    selector: w477 -> [_ w493]
                    tunnel: w476 -> [_ w494]
                    frame No Error {
                    }
                    frame Error {
                      n178 = call <resource>:"GOOP_DebugLogger.vi"("error in (no error)"=w493, "State"=w494) -> ()  [unwired: 7 in, 3 out]
                    }
                  }
                  n179 = Match Pattern(string=w476, regular expression="[.][cC][tT][lLtT]$") -> (offset past match=w485:i32)  [unwired: 4 out]
                  n180 = case shown="6100" w482 {
                    tunnel: w483 -> [_ _ w504 _]
                    tunnel: w477 -> [w499 w500 _ w508]
                    tunnel: [w499 w500 w502 w508] -> w481
                    tunnel: w480 -> [_ _ w502 _]
                    tunnel: w479 -> [_ _ _ w507]
                    tunnel: [_ _ _ w506] -> w478
                    frame 6100 {
                    }
                    frame Default {
                    }
                    frame 1..6099, 6101..6999, 7001.. {
                      n181 = Format Into String(format string="WARNING\nClass: %s\nCould not be completely analysed.\nThis class might have been removed from the current project.", w504) -> (resulting string=w503:string)  [unwired: 2 in, 1 out]
                      n182 = One Button Dialog(message=w503) -> ()  [unwired: 2 out]
                    }
                    frame 7000 {
                      n183 = Format Into String(format string="This class: %s could not be found in the current project.", w507) -> (resulting string=w510:string)  [unwired: 2 in, 1 out]
                      n184 = One Button Dialog(message=w510, button name ("OK")="Abort") -> (true=w506:bool)
                    }
                  }
                  n185 = case shown="-1" w485 {
                    tunnel: w484 -> [_ w498]
                    tunnel: w488 -> [w495 w497]
                    tunnel: [w495 w496] -> w487
                    frame 0, Default {
                    }
                    frame -1 {
                      n186 = Build Array (concatenate)(w497, w498) -> (w496:T7[])
                    }
                  }
                  n187 = Build Array (concatenate)(w492, w490) -> (w491:T3[])
                }
              }
              n188 = call <resource>:"UMLEditor ControlBusyDialog.vi"("I-Value"=w420, "Action(SendStatusMessage)"=UMLEditor_BusyDialogAction."Send_I-Value") -> ()  [unwired: 2 in, 16 out]
              n189 = Unbundle By Name(w445) -> ("baseClasses"=w453:path[], "compAggClasses"=w452:path[], "aggClasses"=w451:path[], "depClasses"=w450:path[])
              n190 = Or(x=w427, y=w425) -> (x .or. y?=w426:bool)
              n191 = Build Array (concatenate)(w439, w453, w452, w451, w450) -> (w454:path[])
              n192 = for {
                shift-right: [w515] -> w434
                shift-left: path[] [] -> [w516]
                tunnel: w454 -> [w513] mode=indexing
                n193 = Search 1D Array(1D array=w516, element=w513) -> (index of element=w514:i32)  [unwired: 1 out]
                n194 = Empty String/Path?(string/path=w513) -> (empty?=w511:bool)
                n195 = Greater Or Equal To 0?(x=w514) -> (x >= 0?=w517:bool)
                n196 = Or(x=w517, y=w511) -> (x .or. y?=w512:bool)
                n197 = case shown="False" w512 {
                  tunnel: w513 -> [w520 _]
                  tunnel: w516 -> [w519 w521]
                  tunnel: [w518 w521] -> w515
                  frame False {
                    n198 = Build Array (concatenate)(w519, w520) -> (w518:path[])
                  }
                  frame True {
                  }
                }
              }
              n199 = Array Size(array=w434) -> (size(s)=w433:i32)
              n200 = case shown="False" w425 {
                tunnel: [w458 w467] -> w435
                tunnel: w421 -> [w456 w466]
                tunnel: w433 -> [_ w465]
                tunnel: w431 -> [w457 w464]
                frame True {
                  n201 = Format Into String(format string="Analysing Class/Type: %d of %d", w456, w456) -> (resulting string=w461:string)  [unwired: 2 in, 1 out]
                  n202 = call <resource>:"UMLEditor ControlBusyDialog.vi"("Title/StatusText"=w461, "error in (no error)"=w457) -> ("error out"=w459:errorcluster)  [unwired: 2 in, 15 out]
                  n203 = call <resource>:"UMLEditor ControlBusyDialog.vi"("error in (no error)"=w459, "Action(SendStatusMessage)"=UMLEditor_BusyDialogAction."GetBusyDialogStatus") -> ("error out"=w458:errorcluster)  [unwired: 2 in, 15 out]
                }
                frame False {
                  n204 = Increment(x=w466) -> (x+1=w471:i32)
                  n205 = Wait (ms)(milliseconds to wait=u32 5) -> ()  [unwired: 1 out]
                  n206 = Format Into String(format string="Analysing Class/Type: %d of %d", w471, w465) -> (resulting string=w470:string)  [unwired: 2 in, 1 out]
                  n207 = call <resource>:"UMLEditor ControlBusyDialog.vi"("Title/StatusText"=w470, "error in (no error)"=w464) -> ("error out"=w468:errorcluster)  [unwired: 2 in, 15 out]
                  n208 = call <resource>:"UMLEditor ControlBusyDialog.vi"("error in (no error)"=w468, "Action(SendStatusMessage)"=UMLEditor_BusyDialogAction."GetBusyDialogStatus") -> ("error out"=w467:errorcluster)  [unwired: 2 in, 15 out]
                }
              }
            }
            n209 = Bundle By Name(cluster=w417, "classInfos"=w412, "TypeDefs"=w414) -> (w418:T10)
            n210 = call <resource>:"GOOP_AnalyseMethodCache.vi"("Actions"=w401, "error in (no error)"=w402) -> ()  [unwired: 7 in, 3 out]
            n211 = call <resource>:"GOOP_AnalyseAttributeCache.vi"("Actions"=w401, "error in (no error)"=w402) -> ()  [unwired: 7 in, 3 out]
          }
          frame "RemoveDublicateTypes" {
            n212 = Unbundle By Name(w525) -> ("TypeDefs"=w527:T3[])
            n213 = for {
              tunnel: w527 -> [w542] mode=indexing
              shift-right: [w541] -> _
              shift-left: path[] [] -> [w540]
              shift-right: [w537] -> w528
              shift-left: i32[] [] -> [w536]
              i -> [w535]
              n214 = Unbundle By Name(w542) -> ("TypeDefPath"=w539:path)
              n215 = Search 1D Array(1D array=w540, element=w539) -> (index of element=w538:i32)  [unwired: 1 out]
              n216 = case shown="-1" w538 {
                tunnel: [w545 w546] -> w537
                tunnel: w536 -> [w544 w546]
                tunnel: w535 -> [w543 _]
                frame 0, Default {
                  n217 = Build Array (concatenate)(w544, w543) -> (w545:i32[])
                }
                frame -1 {
                }
              }
              n218 = Build Array (concatenate)(w540, w539) -> (w541:path[])
            }
            n219 = Reverse 1D Array(array=w528) -> (reversed array=w526:i32[])
            n220 = for {
              shift-right: [w533] -> w524
              shift-left: w527 -> [w534]
              tunnel: w526 -> [w532] mode=indexing
              n221 = Delete From Array(array=w534, index=w532) -> (array with subset deleted=w533:T3[])  [unwired: 1 in, 1 out]
            }
            n222 = Bundle By Name(cluster=w525, "TypeDefs"=w524) -> (w523:T10)
          }
          frame "RemoveClassDependenciesDueToInheritance" {
            n223 = Unbundle By Name(w555) -> ("classInfos"=w552:T7[])
            n224 = for {
              tunnel: w552 -> [w560] mode=indexing
              tunnel: w552 -> [w576] mode=indexing
              tunnel: w552 -> [w574]
              tunnel: w552 -> [w562]
              tunnel: [w566] -> w551 mode=indexing
              n225 = Unbundle By Name(w576) -> ("baseClasses"=w563:path[])
              n226 = Unbundle By Name(w560) -> ("noOfAgg"=w559:i32[])
              n227 = Unbundle By Name(w560) -> ("depClasses"=w571:path[], "aggClasses"=w572:path[], "compAggClasses"=w575:path[])
              n228 = for {
                tunnel: w575 -> [w611] mode=indexing
                tunnel: w574 -> [w610]
                shift-right: [w608] -> w570
                shift-left: path[] [] -> [w607]
                n229 = call <resource>:"ReversedEngineering GetInheritanceClasses.vi"("classInfos"=w610, "classPath"=w611) -> ("baseClasses"=w609:path[])  [unwired: 17 out]
                n230 = Build Array (concatenate)(w609, w607) -> (w608:path[])
              }
              n231 = call <resource>:"ReversedEngineering RemoveThesePathes.vi"("classesIn"=w572, "removeThese"=w570) -> ("classesOut"=w564:path[], "Removed(Index-1*n)"=w561:i32[])  [unwired: 16 out]
              n232 = for {
                tunnel: w561 -> [w580] mode=indexing
                shift-right: [w578] -> w558
                shift-left: w559 -> [w577]
                n233 = Delete From Array(array=w577, length=1, index=w580) -> (array with subset deleted=w578:i32[])  [unwired: 1 out]
              }
              n234 = for {
                tunnel: w564 -> [w586] mode=indexing
                tunnel: w564 -> [w594]
                shift-right: [w589] -> w567
                shift-left: path[] [] -> [w590]
                tunnel: w562 -> [w585]
                shift-right: [w581] -> w556
                shift-left: i32[] [] -> [w583]
                tunnel: w558 -> [w582] mode=indexing
                i -> [w593]
                n235 = call <resource>:"ReversedEngineering GetInheritanceClasses.vi"("classInfos"=w585, "classPath"=w586) -> ("baseClasses"=w584:path[])  [unwired: 17 out]
                n236 = Delete From Array(array=w594, length=1, index=w593) -> (array with subset deleted=w591:path[])  [unwired: 1 out]
                n237 = for {
                  tunnel: w591 -> [w604]
                  tunnel: w584 -> [w605] mode=indexing
                  tunnel: [w603] -> w588 mode=indexing
                  n238 = Search 1D Array(1D array=w604, element=w605) -> (index of element=w606:i32)  [unwired: 1 out]
                  n239 = Greater Or Equal To 0?(x=w606) -> (x >= 0?=w603:bool)
                }
                n240 = Or Array Elements(Boolean array=w588) -> (logical OR=w587:bool)
                n241 = case shown="False" w587 {
                  tunnel: w590 -> [w600 w602]
                  tunnel: [w599 w602] -> w589
                  tunnel: w586 -> [w598 _]
                  tunnel: w583 -> [w597 w601]
                  tunnel: w582 -> [w596 _]
                  tunnel: [w595 w601] -> w581
                  frame False {
                    n242 = Build Array (concatenate)(w597, w596) -> (w595:i32[])
                    n243 = Build Array (concatenate)(w600, w598) -> (w599:path[])
                  }
                  frame True {
                  }
                }
              }
              n244 = call <resource>:"ReversedEngineering RemoveThesePathes.vi"("classesIn"=w571, "removeThese"=w570) -> ("classesOut"=w569:path[])  [unwired: 17 out]
              n245 = call <resource>:"ReversedEngineering RemoveThesePathes.vi"("classesIn"=w569, "removeThese"=w563) -> ("classesOut"=w565:path[])  [unwired: 17 out]
              n246 = Bundle By Name(cluster=w560, "depClasses"=w565, "aggClasses"=w567, "noOfAgg"=w556) -> (w566:T7)
            }
            n247 = Bundle By Name(cluster=w555, "classInfos"=w551) -> (w554:T10)
            n248 = Select(t="AddApplicationNodes" ("y"), s=w547, f="Exit" ("y")) -> (s? t:f=w549:string)
          }
          frame "AddApplicationNodes" {
            n249 = Unbundle By Name(w622) -> ("classInfos"=w619:T7[], "dependencyClassPath"=w617:path[], "TopVIPath"=w616:path)
            n250 = Empty String/Path?(string/path=w616) -> (empty?=w615:bool)
            n251 = Bundle By Name(cluster=T7 {"classPath"=path "", "inherits"=FALSE, "baseClasses"=[], "compAggClasses"=[], "noOfCompObj"=[], "aggClasses"=[], "noOfAgg"=[], "depClasses"=[], "methods"=[], "methodPuplic"=[], "objectAttrib"=[], "classAttrib"=[], "ClassDesc"="", "DependencyDetails"=[]} ("classInfo"), "ClassDesc"="<<APPLICATION>>") -> (w613:T7)
            n252 = case shown="False" w615 {
              tunnel: w619 -> [w629 w630]
              tunnel: [w628 w630] -> w618
              tunnel: w613 -> [w627 _]
              tunnel: w617 -> [w626 _]
              tunnel: w616 -> [w624 _]
              frame False {
                n253 = Bundle By Name(cluster=w627, "depClasses"=w626, "classPath"=w624) -> (w625:T7)
                n254 = Build Array (concatenate)(w625, w629) -> (w628:T7[])
              }
              frame True {
              }
            }
            n255 = Bundle By Name(cluster=w622, "classInfos"=w618) -> (w621:T10)
          }
          frame "Error", Default {
          }
        }
        n256 = Unbundle By Name(w67) -> ("status"=w63:bool)
        n257 = Equal?(x=w66, y="Exit") -> (x = y?=w64:bool)
        n258 = Or(x=w64, y=w63) -> (x .or. y?=w62:bool)
      }
    }
    frame Error {
    }
  }
  n259 = Unbundle By Name(w26) -> ("TypeDefs"=w14:T3[], "classInfos"=w13:T7[], "VIRef"=w22:refnum<vi>[])
  n260 = call <resource>:"Error_ClearError.vi"("codes"=i32[] [6100, 7000], "error in (no error)"=w17) -> ("Cleared?"=w15:bool, "error out"=→"error out":errorcluster)  [unwired: 3 in, 13 out]
  "Cancelled" <- w15
  n261 = call <resource>:"ReversedEngineering ViCachMemory.vi"("ViRef-Array"=w22) -> ()  [unwired: 3 in, 16 out]
  n262 = case shown="True" w15 {
    tunnel: w14 -> [w636 _]
    tunnel: w13 -> [w635 _]
    tunnel: [w636 _] -> w12
    tunnel: [w635 _] -> w11
    frame False {
    }
    frame True {
    }
  }
  "classInfos" <- w11
  "TypeDefs" <- w12
